vi "AI_OneBufferedAI_USB4704 polymorph v3.vi"() -> ()   [LabVIEW 2013]
uses:
  <vilib>/Platform/TimedLoop/XDataNode/timing_clust.ctl
  <vilib>/Platform/TimedLoop/XDataNode/nitl_modes.ctl
  <vilib>/Platform/TimedLoop/XDataNode/wakeup.ctl
  <userlib>/DAQNavi Polymorphic VI/create/DAQNavi Create Channel(AI-Voltage).vi
  <userlib>/DAQNavi Polymorphic VI/configure/timing/DAQNavi Timing(Convert Clock).vi
  <userlib>/DAQNavi Polymorphic VI/read/DAQNavi Read (Analog 1D Wfm NChan NSamp).vi
  <vilib>/platform/TimedLoop/XDataNode/XDataNode.xnode
  <vilib>/Platform/TimedLoop/XDataNode/XDNodeRunTimeDep.lvlib
panel:
  out "Test":timestamp
  out "Start":timestamp
  out "error out":errorcluster
  out "value range":string="+/- 5 V" caption="property value"
  in  "samples per channel":i32=1000
  in  "convert clock rate":dbl=1000.0
  out "physical channels":string="DemoDevice,BID#0/ai0:1" caption="property value"
  in  "Stop Button":bool
  out "loop":bool
  out "Waveform Graph":waveform(dbl)[](graph)
  in  "number of samples per channel to read":u32=1000
  # "Please modify physical channels and value range in Channel Parameters\nthrough DAQNavi Property Assistant VI  in block diagram."
  # "Channel Parameters"
  # "Timing Parameters"
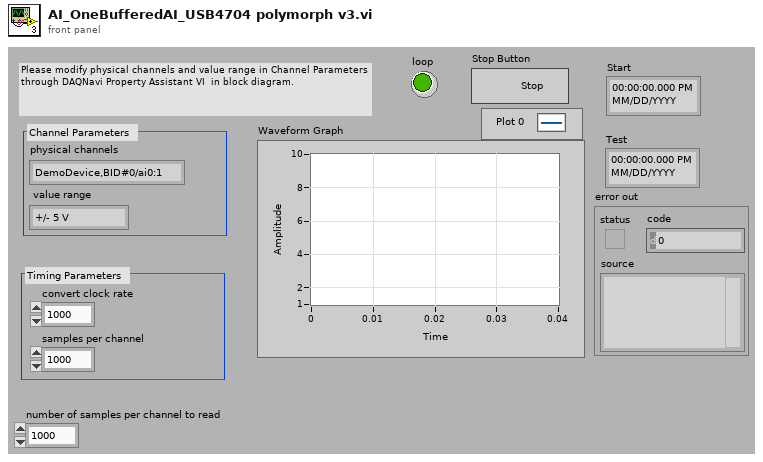
[diagram p1: front panel]
types:
  T1 = typedef "XDNodeRunTimeDep.lvlib/timing_clust.ctl" = cluster{"Expected End [f-1]":u64, "Actual End [f-1]":u64, "Finished Late? [f-1]":bool, "Expected End [i-1]":u64, "Actual End [i-1]":u64, "Finished Late? [i-1]":bool, "Expected Start [i]":u64, "Actual Start [i]":u64, "Expected Start [f]":u64, "Actual Start [f]":u64, "Source Name":string, "Structure Name":string, "Period":i64, "Deadline":i64, "Offset":i64, "Start":i64, "Priority":i32, "Timeout":i32, "Mode":T2, "Wakeup Reason":T3, "Error":errorcluster, "Source Type":string, "Secondary Source Type":string, "Global End Time":u64, "Global Start Time":u64, "Frame Duration":u64, "Iteration Duration":u64, "Assigned CPU":i32, "I/O Scan Engine Mode":u32}
  T2 = typedef "XDNodeRunTimeDep.lvlib/nitl_modes.ctl" = enum32{"No Change", "Process missed periods, maintain original phase", "Discard missed periods, maintain original phase", "Process missed periods, ignore original phase", "Discard missed periods, ignore original phase"}
  T3 = typedef "XDNodeRunTimeDep.lvlib/wakeup.ctl" = enum32{"Normal", "Aborted", "Asynchronous wakeup", "Timing source error", "Timed loop error", "Timeout"}
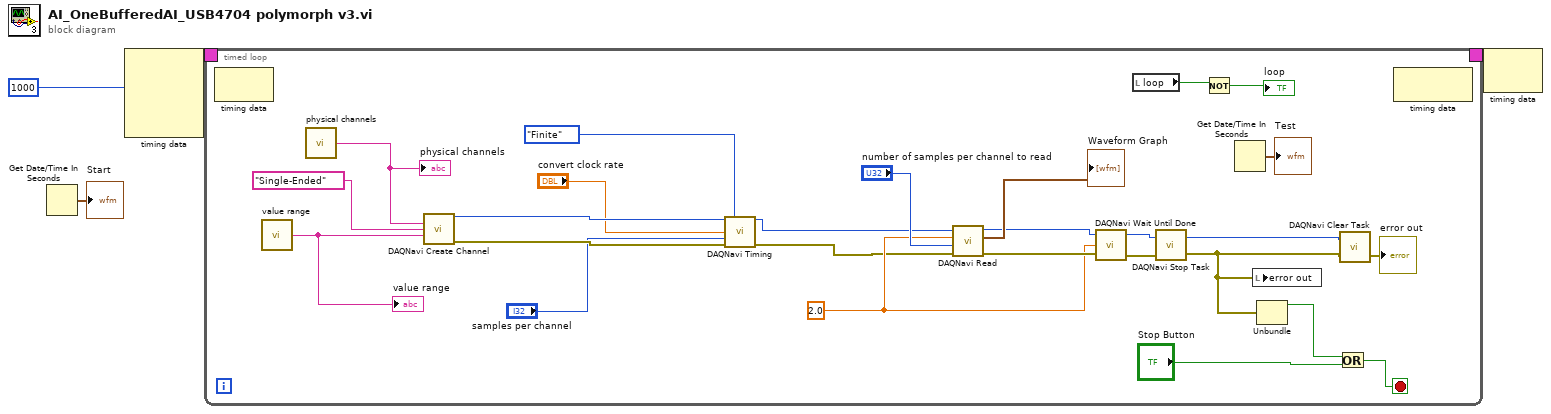
[diagram p0: block diagram]
diagram:
  n1 = Get Date/Time In Seconds() -> (seconds since 1Jan1904=→"Start":timestamp)
  n2 = node-c288(1000) -> (w4:T1)  [unwired: 3 in]
  n3 = timed-loop {
    timing: w4 -> [_]
    timing-out: [_] -> w3
    stop <- w24 stop-if-true
    w19 = 2.0 ("timeToWait")
    n4 = node-c288() -> ()  [unwired: 1 in, 1 out]
    n5 = call "value range"() -> ("property value"=w10:string)  [unwired: 1 out]
    "value range" <- w10
    n6 = call "physical channels"() -> ("property value"=w11:string)  [unwired: 1 out]
    "physical channels" <- w11
    n7 = call-poly <userlib>:"DAQNavi Create Channel.vi"("physical channels"=w11, "signal type"="Single-Ended", "value range"=w10) -> ("task out"=w16:i32, "error out"=w15:errorcluster)  [unwired: 2 in, 9 out]
    n8 = call-poly <userlib>:"DAQNavi Timing.vi"("task in"=w16, "sample mode"=enum16{"Finite", "Continuous"}."Finite", "rate"="convert clock rate", "samples per channel"="samples per channel", "error in (no error)"=w15) -> ("task out"=w6:i32, "error out"=w5:errorcluster)  [unwired: 1 in, 8 out]
    n9 = call-poly <userlib>:"DAQNavi Read.vi"("error in (no error)"=w5, "number of samples per channel to read"="number of samples per channel to read", "timeout"=w19, "task in"=w6) -> ("error out"=w22:errorcluster, "data"=→"Waveform Graph":waveform(dbl)[], "task out"=w23:i32)  [unwired: 5 out]
    n10 = call <userlib>:"DAQNavi Wait Until Done.vi"("error in (no error)"=w22, "timeToWait"=w19, "task in"=w23) -> ("error out"=w20:errorcluster, "task out"=w21:i32)  [unwired: 1 in]
    n11 = local read "loop"() -> (w28:bool)
    n12 = call <userlib>:"DAQNavi Stop Task.vi"("error in (no error)"=w20, "task in"=w21) -> ("error out"=w7:errorcluster, "task out"=w8:i32)
    n13 = Not(x=w28) -> (.not. x?=→"loop":bool)
    n14 = Get Date/Time In Seconds() -> (seconds since 1Jan1904=→"Test":timestamp)
    n15 = local write "error out"(w7) -> ()
    n16 = Unbundle(w7) -> ("status"=w25:bool)  [unwired: 2 out]
    n17 = Or(x=w25, y="Stop Button") -> (x .or. y?=w24:bool)
    n18 = call <userlib>:"DAQNavi Clear Task.vi"("error in (no error)"=w7, "task in"=w8) -> ("error out"=→"error out":errorcluster)  [unwired: 1 out]
    n19 = node-c288() -> ()  [unwired: 1 in, 1 out]
  }
  n20 = node-c288(w3) -> ()  [unwired: 1 out]
